vi "IMAQdx Configure Ring Acquisition.vi"(7 "Mode":T2=enum."Continuous", 8 "error in":errorcluster, 10 "Images":T1[](array[typedef]), 11 "Session In":T3) -> (0 "error out":errorcluster, 2 "Images Out":T1[](array[typedef]), 3 "Session Out":T3)   [LabVIEW 2020, in "NI_Vision_Acquisition_Software.lvlib"]
doc: "Configures a ring acquisition. A ring acquisition is an acquisition in which the image is acquired directly into the images in the <B>Images</B> array."
uses:
  NI_Vision_Acquisition_Software.lvlib
  IMAQdx.ctl
  IMAQdx Acquisition Mode.ctl
  IMAQ Image.ctl
  niimaqdx.dll
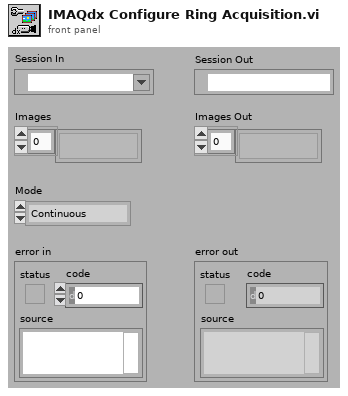
[diagram p1: front panel]
types:
  T1 = typedef "IMAQ Image.ctl" = refnum<image>
  T2 = typedef "NI_Vision_Acquisition_Software.lvlib/IMAQdx Acquisition Mode.ctl" = enum32{"One Shot", "Continuous"}
  T3 = typedef "IMAQdx.ctl" = refnum<k21>
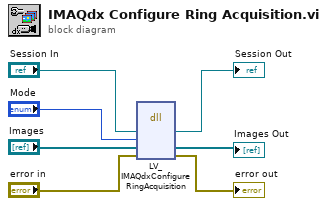
[diagram p0: block diagram]
diagram:
  n1 = dll-call lib="niimaqdx.dll" fn="LV_IMAQdxConfigureRingAcquisition"("refnum"="Session In", "continuous"="Mode", "images"="Images", "error"="error in") -> ("refnum"=→"Session Out":T3, "images"=→"Images Out":T1[], "error"=→"error out":errorcluster)  [unwired: 5 in, 2 out]
